vi "Unlock DB.vi"(8 "error in (no error)":errorcluster, 9 "SQLite DB":refnum<class "Connection.lvclass">, 11 "SQLite in":refnum<class "SQLite.lvclass">) -> (0 "error out":errorcluster, 3 "SQLite out":refnum<class "SQLite.lvclass">)   [LabVIEW 2020, in "Summer of LabVIEW.lvlib" / "SQLite.lvclass"]
uses:
  SQLite.lvclass
  <vilib>/drjdpowell/SQLite Library/SQL Connection/Connection.lvclass
  SQLite.lvclass/SQLite.ctl
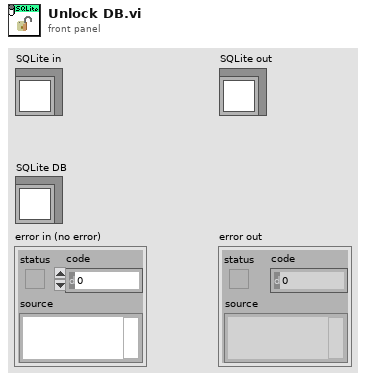
[diagram p1: front panel]
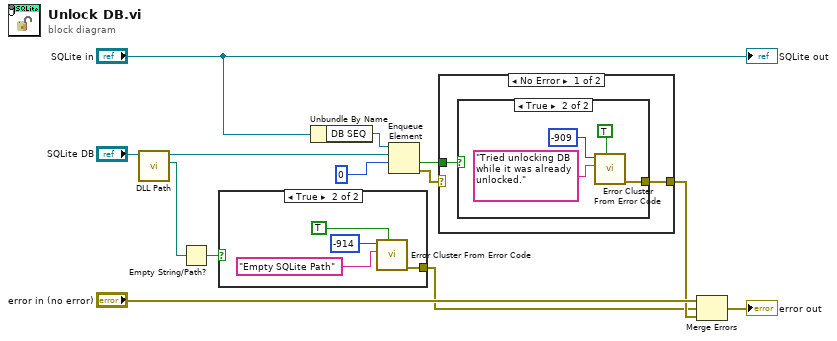
[diagram p0: block diagram]
diagram:
  n1 = call <vilib>:"DLL Path.vi"("Connection in"="SQLite DB") -> ("SQLite dll"=w3:path, "Connection out"=w4:refnum<class "Connection.lvclass">)  [unwired: 8 in, 1 out]
  n2 = Empty String/Path?(string/path=w3) -> (empty?=w2:bool)
  n3 = case shown="True" w2 {
    tunnel: [_ w14] -> w1
    frame False {
    }
    frame True {
      n4 = call <vilib>:"Error Cluster From Error Code.vi"("show call chain? (False)"=TRUE, "error message (\"\")"="Empty SQLite Path" ("error message (\"\")"), "error code (0)"=-914) -> ("error out"=w14:errorcluster)  [unwired: 6 in]
    }
  }
  n5 = Unbundle By Name("SQLite in") -> ("DB SEQ"=w11:refnum<queue>)
  n6 = Enqueue Element(queue=w11, element=w4, timeout in ms (-1)=0) -> (timed out?=w9:bool, error out=w8:errorcluster)  [unwired: 1 in, 1 out]
  n7 = case shown="No Error" w8 {
    selector: w8 -> [_ w24]
    tunnel: w9 -> [w19 _]
    tunnel: [w18 w24] -> w6
    frame No Error {
      n8 = case shown="True" w19 {
        tunnel: [_ w23] -> w18
        frame False {
        }
        frame True {
          n9 = call <vilib>:"Error Cluster From Error Code.vi"("show call chain? (False)"=TRUE, "error message (\"\")"="Tried unlocking DB while it was already unlocked." ("error message (\"\")"), "error code (0)"=-909) -> ("error out"=w23:errorcluster)  [unwired: 6 in]
        }
      }
    }
    frame Error {
    }
  }
  n10 = Merge Errors("error in (no error)", w1, w6) -> (→"error out":errorcluster)
  "SQLite out" <- "SQLite in"
